vi "New.vi"(8 "error in (no error)":errorcluster, 11 "reference in":refnum<class "SMO_TestSuite.lvclass">) -> (0 "error out":errorcluster, 3 "reference out":refnum<class "SMO_TestSuite.lvclass">)   [LabVIEW 2013, in "SMO_TestSuite.lvclass"]
uses:
  SMO_TestSuite.lvclass
  <vilib>/addons/_JKI Toolkits/VI Tester/TestCase.llb/TestCase.lvclass
  SMO_TestCase/SMO_TestCase.lvclass
  SMO.UI_TestCase/SMO.UI_TestCase.lvclass
  SMO_TestSuite.lvclass/SMO_TestSuite.ctl
  <vilib>/addons/_JKI Toolkits/VI Tester/TestSuite.llb/TestSuite.lvclass
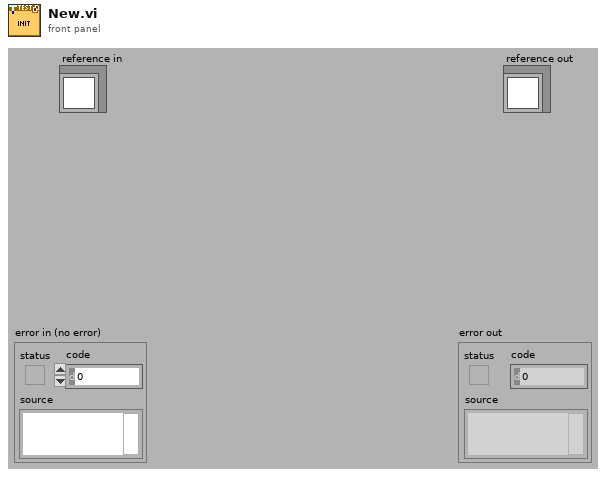
[diagram p1: front panel]
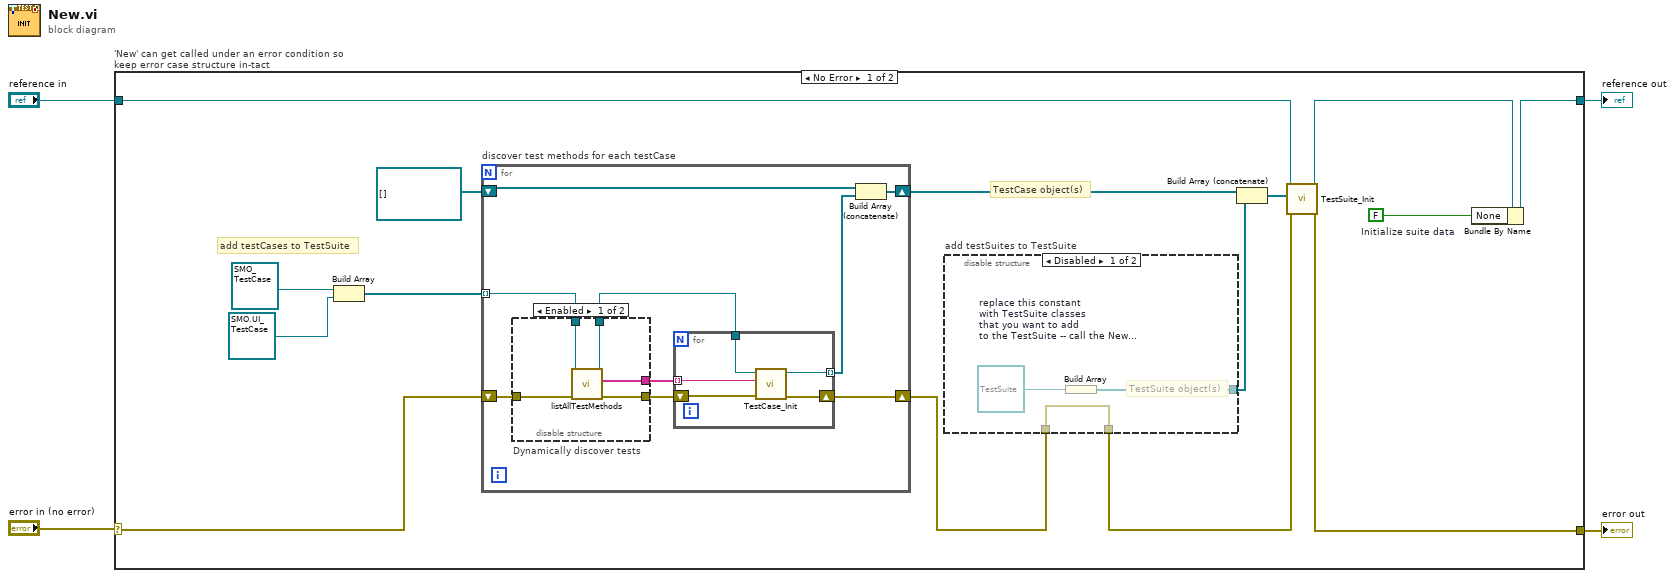
[diagram p0: block diagram]
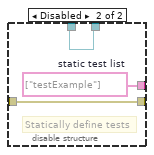
[diagram p2: hidden frame]
diagram:
  n1 = case "'New' can get called under an error condition so keep error case structure in-tact" shown="No Error" "error in (no error)" {
    selector: "error in (no error)" -> [w13 w46]
    tunnel: [w19 w47] -> w4
    tunnel: "reference in" -> [w14 w47]
    tunnel: [w16 w46] -> w1
    frame No Error {
      w18 = FALSE  # Initialize suite data
      # "TestCase object(s)"
      # "add testCases to TestSuite"
      n2 = Build Array(refnum<class "SMO_TestCase.lvclass"> refnum ("SMO_TestCase.lvclass"), refnum<class "SMO.UI_TestCase.lvclass"> refnum ("SMO.UI_TestCase.lvclass")) -> (w15:refnum<class "TestCase.lvclass">[])
      n3 = for "discover test methods for each testCase" {
        shift-right: [w28] -> w8
        shift-left: w13 -> [w24]
        tunnel: w15 -> [w21] mode=indexing
        shift-right: [w25] -> w12
        shift-left: refnum<class "TestCase.lvclass">[] [] -> [w26]
        n4 = disable-structure "Dynamically discover tests" shown="Enabled" {
          disable-tunnel: w24 -> [w33 w34]
          disable-tunnel: [w32 w34] -> w23
          disable-tunnel: [w31 w35] -> w22
          disable-tunnel: w21 -> [w30 w36]
          disable-tunnel: [w29 w36] -> w20
          frame Enabled {
            n5 = call-dynamic "listAllTestMethods.vi"("error in (no error)"=w33, "TestCase in"=w30) -> ("error out"=w32:errorcluster, "test methods"=w31:string[], "TestCase out"=w29:refnum<class "TestCase.lvclass">)  [unwired: 7 in]
          }
          frame Disabled {
            w35 = string[] ["testExample"]  # static test list
            # "Statically define tests"
          }
        }
        n6 = for {
          tunnel: w20 -> [w37]
          tunnel: w22 -> [w41] mode=indexing
          shift-right: [w39] -> w28
          shift-left: w23 -> [w40]
          tunnel: [w38] -> w27 mode=indexing
          n7 = call <vilib>:"TestCase_Init.vi"("error in (no error)"=w40, "methodName (\"runTest\")"=w41, "TestCase in"=w37) -> ("error out"=w39:errorcluster, "TestCase out"=w38:refnum<class "TestCase.lvclass">)  [unwired: 7 in]
        }
        n8 = Build Array (concatenate)(w26, w27) -> (w25:refnum<class "TestCase.lvclass">[])
      }
      n9 = disable-structure "add testSuites to TestSuite" shown="Disabled" {
        disable-tunnel: [w42 _] -> w10
        disable-tunnel: [w44 w45] -> w9
        disable-tunnel: w8 -> [w44 w45]
        frame Disabled {
          w43 = refnum<class "TestSuite.lvclass"> refnum  # replace this constant with TestSuite classes that you want to add to the TestSuite -- call the New method for each TestSuite prior to adding it to this TestSuite
          # "TestSuite object(s)"
          n10 = Build Array(w43) -> (w42:refnum<class "TestSuite.lvclass">[])
        }
        frame Enabled {
          # "by default, no TestSuites are defined\nas members of a TestSuite"
        }
      }
      n11 = Build Array (concatenate)(w12, w10) -> (w11:refnum<class>[])
      n12 = call <vilib>:"TestSuite_Init.vi"("error in (no error)"=w9, "tests (none)"=w11, "TestSuite in"=w14) -> ("error out"=w16:errorcluster, "TestSuite out"=w17:refnum<class "SMO_TestSuite.lvclass">)  [unwired: 7 in]
      n13 = Bundle By Name(cluster=w17, "None"=w18) -> (w19:refnum<class "SMO_TestSuite.lvclass">)
    }
    frame Error {
    }
  }
  "reference out" <- w4
  "error out" <- w1
